vi "Untitled 4.vi"() -> ()   [LabVIEW 2014]
panel:
  out "Triggered":bool
  in  "Threshold":dbl
  in  "Slide Control":dbl(slide) scale=0.0..10.0
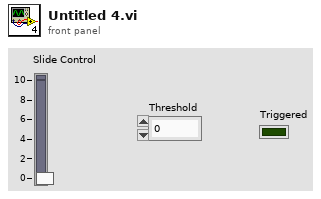
[diagram p1: front panel]
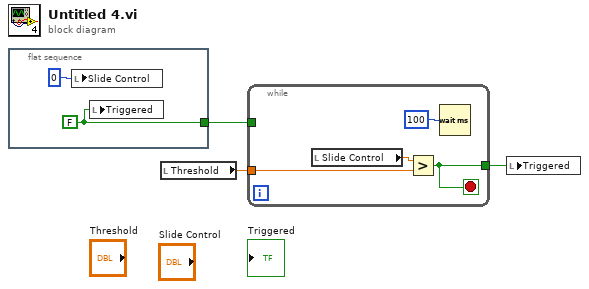
[diagram p0: block diagram]
diagram:
  n1 = flat-sequence {
    tunnel: [w4] -> w3
    frame #0 {
      w4 = FALSE
      n2 = local write "Slide Control"(0) -> ()
      n3 = local write "Triggered"(w4) -> ()
    }
  }
  n4 = local read "Threshold"() -> (w1:dbl)
  n5 = while {
    tunnel: w3 -> [_]
    tunnel: [w7] -> w2
    tunnel: w1 -> [w9]
    stop <- w7 stop-if-true
    n6 = local read "Slide Control"() -> (w8:dbl)
    n7 = Greater?(x=w8, y=w9) -> (0:w7:bool)
    n8 = Wait (ms)(milliseconds to wait=100) -> ()  [unwired: 1 out]
  }
  n9 = local write "Triggered"(w2) -> ()
